vi "EX1.vi"(8 "str":string="Номер партии проверяемых пластин", 11 "Panel":T1) -> ()   [LabVIEW 2015]
uses:
  <vilib>/Utility/miscctls.llb/LVRectTypeDef.ctl
panel:
  out "String":string
  in  "stop":bool
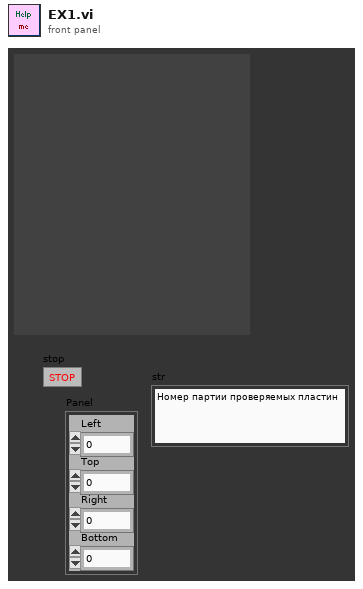
[diagram p1: front panel]
types:
  T1 = typedef "LVRectTypeDef.ctl" = cluster{"Left":i16, "Top":i16, "Right":i16, "Bottom":i16}
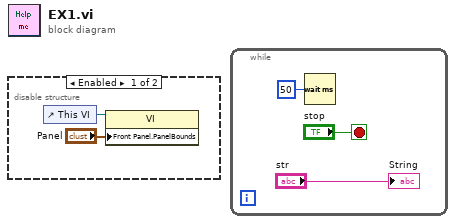
[diagram p0: block diagram]
diagram:
  n1 = disable-structure shown="Enabled" {
    frame Enabled {
      n2 = control-ref of="This VI"() -> (w2:refnum<vi>)
      n3 = property class="VI"(reference=w2, "Front Panel.PanelBounds"="Panel") -> ()  [unwired: 1 in, 2 out]
    }
    frame Disabled {
    }
  }
  n4 = while {
    stop <- "stop" stop-if-true
    n5 = Wait (ms)(milliseconds to wait=u32 50) -> ()  [unwired: 1 out]
    "String" <- "str"
  }
